vi "Get Measurement Details.vi"(8 "error in":errorcluster) -> (0 "error out":errorcluster, 2 "Service ID":string, 3 "measurement_details":T1)   [LabVIEW 2020, in "LineRegulation.lvlib"]
uses:
  LineRegulation.lvlib
  RPC Messages/ni_measurements_v1_MeasurementDetails.ctl
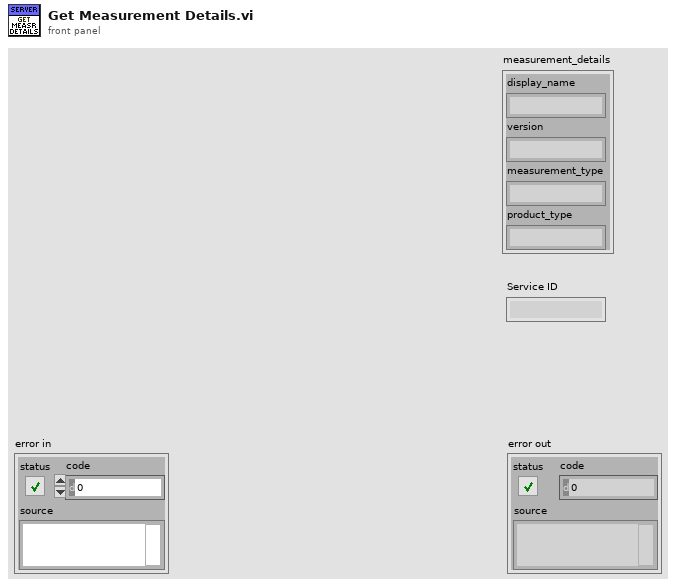
[diagram p1: front panel]
types:
  T1 = typedef "LineRegulation.lvlib/ni_measurements_v1_MeasurementDetails.ctl" = cluster{"display_name":string, "version":string, "measurement_type":string, "product_type":string}
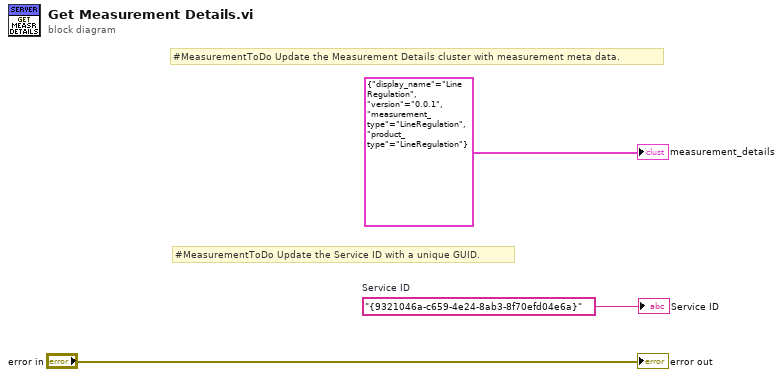
[diagram p0: block diagram]
diagram:
  w1 = "{9321046a-c659-4e24-8ab3-8f70efd04e6a}"  # Service ID
  # "#MeasurementToDo Update the Service ID with a unique GUID."
  # "#MeasurementToDo Update the Measurement Details cluster with measurement meta data."
  "error out" <- "error in"
  "measurement_details" <- T1 {"display_name"="Line Regulation", "version"="0.0.1", "measurement_type"="LineRegulation", "product_type"="LineRegulation"} ("ni_measurements_v1_MeasurementDetails")
  "Service ID" <- w1
